vi "DAQ Channel Dlg_V0.vi"(7 "DAQ Sample Rate (S/s)":i32=100, 9 "AO Channel":enum16{"0", "1"}(ring), 10 "Device Name":tag) -> (2 "Chl Infor":variant)   [LabVIEW 2021]
doc: "This vi helps to check if channels are in valid range and pass Channel Information out as a variant."
uses:
  Controls/Channel Selection/Volt Chl.ctl
panel:
  in  "OK Button":bool
  in  "Channel Array":T1(array[cluster])=[{"Ch"=0, "Desc"="Channel 0:", "Scale"=1.0, "Offset"=0.0, "Selected"=FALSE}, {"Ch"=1, "Desc"="Channel 1:", "Scale"=1.0, "Offset"=0.0, "Selected"=FALSE}, {"Ch"=2, "Desc"="Channel 2:", "Scale"=1.0, "Offset"=0.0, "Selected"=FALSE}, {"Ch"=3, "Desc"="Channel 3:", "Scale"=1.0, "Offset"=0.0, "Selected"=FALSE}, {"Ch"=4, "Desc"="Channel 4:", "Scale"=1.0, "Offset"=0.0, "Selected"=FALSE}, {"Ch"=5, "Desc"="Channel 5:", "Scale"=1.0, "Offset"=0.0, "Selected"=FALSE}, {"Ch"=6, "Desc"="Channel 6:", "Scale"=1.0, "Offset"=0.0, "Selected"=FALSE}, {"Ch"=7, "Desc"="Channel 7:", "Scale"=1.0, "Offset"=0.0, "Selected"=FALSE}, {"Ch"=8, "Desc"="", "Scale"=1.0, "Offset"=0.0, "Selected"=FALSE}, {"Ch"=9, "Desc"="", "Scale"=1.0, "Offset"=0.0, "Selected"=FALSE}, {"Ch"=10, "Desc"="", "Scale"=1.0, "Offset"=0.0, "Selected"=FALSE}, {"Ch"=11, "Desc"="", "Scale"=1.0, "Offset"=0.0, "Selected"=FALSE}, {"Ch"=12, "Desc"="", "Scale"=1.0, "Offset"=0.0, "Selected"=FALSE}, {"Ch"=13, "Desc"="", "Scale"=1.0, "Offset"=0.0, "Selected"=FALSE}, {"Ch"=14, "Desc"="", "Scale"=1.0, "Offset"=0.0, "Selected"=FALSE}, {"Ch"=15, "Desc"="", "Scale"=1.0, "Offset"=0.0, "Selected"=FALSE}]
  # "Ch"
  # "Description"
  # "Scale"
  # "Offset"
  # "Select Ch"
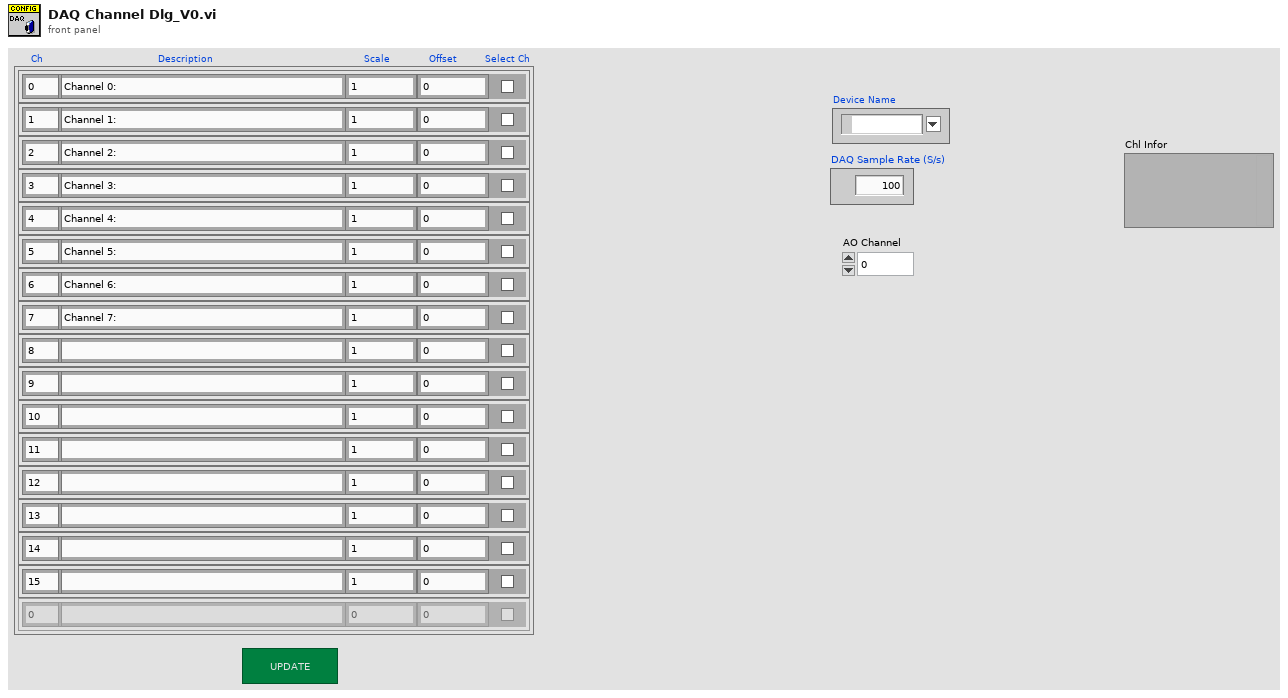
[diagram p1: front panel]
types:
  T1 = cluster{"Ch":i32, "Desc":string, "Scale":dbl, "Offset":dbl, "Selected":bool}[]
  T2 = typedef "Volt Chl.ctl" = cluster{"Index":i32[], "Chl Name":string[], "Scale":dbl[], "Offset":dbl[], "Sample Rate":i32, "Device Name":tag, "Channel":tag, "AO Channel":tag}
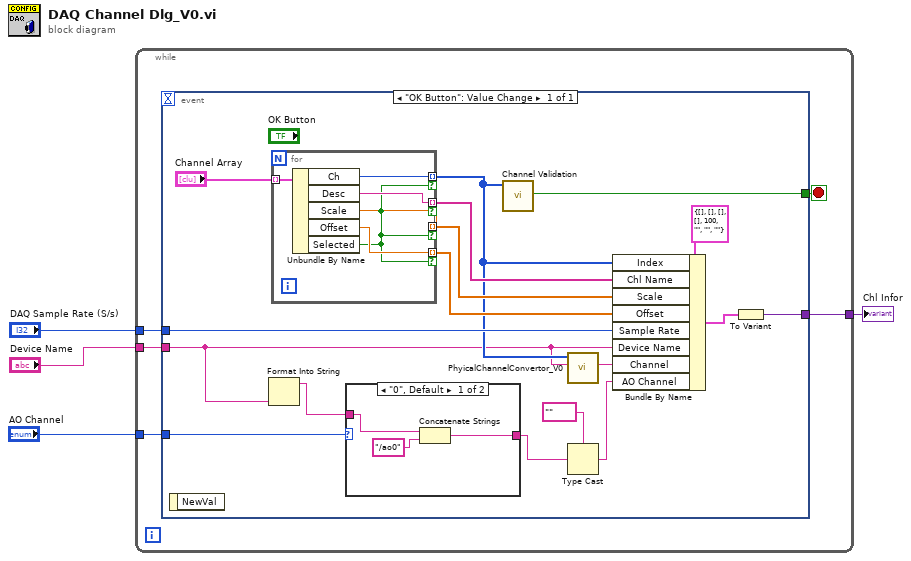
[diagram p0: block diagram]
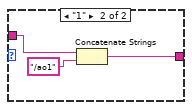
[diagram p2: hidden frame]
diagram:
  n1 = while {
    tunnel: "DAQ Sample Rate (S/s)" -> [w8]
    tunnel: "Device Name" -> [w7]
    tunnel: [w6] -> w2
    tunnel: "AO Channel" -> [w5]
    stop <- w9 stop-if-true
    n2 = event shown="[0] \"OK Button\": Value Change" {
      selector: _ -> [_]
      dyn-events: _ -> [_]
      timeout: _ -> [_]
      tunnel: [w22] -> w9
      tunnel: w8 -> [w21]
      tunnel: w7 -> [w14]
      tunnel: [w17] -> w6
      tunnel: w5 -> [w13]
      event "OK Button": Value Change {
        n3 = event-data() -> ()  [unwired: 1 in, 1 out]
        n4 = Format Into String(w14) -> (resulting string=w15:string)  [unwired: 3 in, 1 out]
        n5 = for {
          tunnel: "Channel Array" -> [w38] mode=indexing
          tunnel: [w37] -> w20 mode=indexing if=w33
          tunnel: [w36] -> w25 mode=indexing if=w33
          tunnel: [w35] -> w24 mode=indexing if=w33
          tunnel: [w34] -> w23 mode=indexing if=w33
          n6 = Unbundle By Name(w38) -> ("Ch"=w37:i32, "Desc"=w36:string, "Scale"=w35:dbl, "Offset"=w34:dbl, "Selected"=w33:bool)
        }
        n7 = case shown="\"0\", Default" w13 {
          tunnel: w15 -> [w29 w32]
          tunnel: [w28 w31] -> w12
          frame "0", Default {
            n8 = Concatenate Strings(w29, "/ao0" ("string")) -> (w28:string)
          }
          frame "1" {
            n9 = Concatenate Strings(w32, "/ao1" ("string")) -> (w31:string)
          }
        }
        n10 = call "Channel Validation.vi"("User Defined Channels"=w20) -> ("Chl Valid?"=w22:bool)  [unwired: 10 in]
        n11 = call "PhyicalChannelConvertor_V0.vi"("Device Name"=w14, "Channel Number Array"=w20) -> ("physical channels"=w19:tag)  [unwired: 9 in]
        n12 = Type Cast(type=tag "" ("physical channels"), x=w12) -> (*(type *) &x=w10:tag)
        n13 = Bundle By Name(cluster=T2 {"Index"=[], "Chl Name"=[], "Scale"=[], "Offset"=[], "Sample Rate"=100, "Device Name"="", "Channel"="", "AO Channel"=""}, "Index"=w20, "Chl Name"=w25, "Scale"=w24, "Offset"=w23, "Sample Rate"=w21, "Device Name"=w14, "Channel"=w19, "AO Channel"=w10) -> (w18:T2)
        n14 = To Variant(anything=w18) -> (Variant=w17:variant)
      }
    }
  }
  "Chl Infor" <- w2
